vi "Listen.vi"(8 "error in (no error)":errorcluster, 10 "timeout in ms (-1)":i32=-1, 11 "input in":refnum<class "input.lvclass">) -> (0 "error out":errorcluster, 1 "timed out?":bool, 2 "Result":refnum<class "result.lvclass">, 3 "input out":refnum<class "input.lvclass">)   [LabVIEW 2015, in "input.lvclass"]
uses:
  input.lvclass
  Result/result.lvclass
  input.lvclass/input.ctl
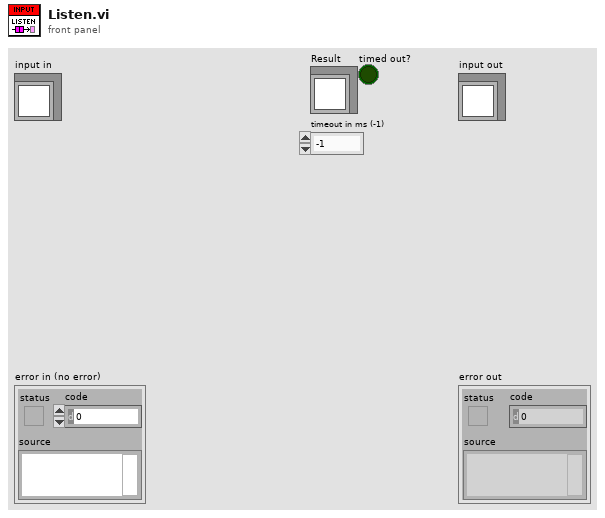
[diagram p1: front panel]
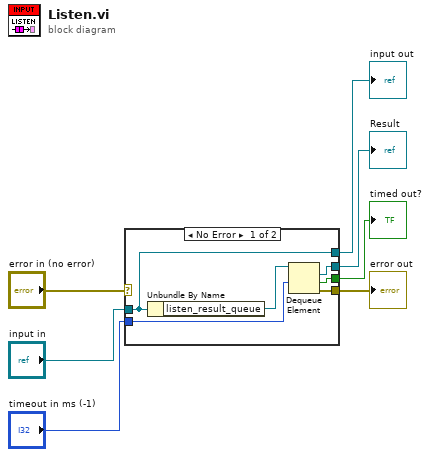
[diagram p0: block diagram]
diagram:
  n1 = case shown="No Error" "error in (no error)" {
    selector: "error in (no error)" -> [_ w15]
    tunnel: [w11 w15] -> w6
    tunnel: [w13 w14] -> w4
    tunnel: "input in" -> [w13 w14]
    tunnel: "timeout in ms (-1)" -> [w10 _]
    tunnel: [w9 _] -> w2
    tunnel: [w8 _] -> w1
    frame No Error {
      n2 = Unbundle By Name(w13) -> ("listen_result_queue"=w12:refnum<queue>)
      n3 = Dequeue Element(queue=w12, timeout in ms (-1)=w10) -> (element=w9:refnum<class "result.lvclass">, timed out?=w8:bool, error out=w11:errorcluster)  [unwired: 1 in, 1 out]
    }
    frame Error {
    }
  }
  "error out" <- w6
  "input out" <- w4
  "Result" <- w2
  "timed out?" <- w1
